vi "Calculation.vi"(4 "Calibration Factor":dbl, 5 "Frequency (Hz)":dbl, 6 "dµ (µg/mm)":dbl, 7 "t < 1.5 s ?":bool, 8 "dL (mm)":dbl, 9 "df (Hz)":dbl, 10 "Wire Linear Density In":dbl, 11 "Wire Length In":dbl) -> (0 "Linear Density (µm/mm)":dbl, 1 "Wire Length (mm)":dbl, 2 "dT (g)":dbl, 3 "Tension (g)":dbl)   [LabVIEW 2018]
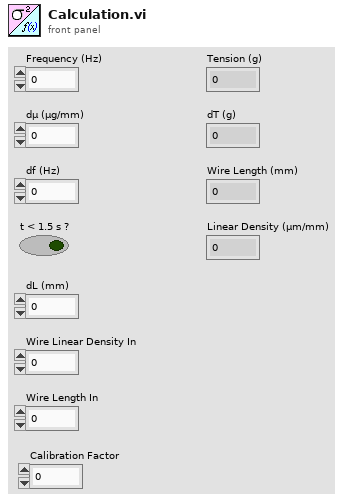
[diagram p1: front panel]
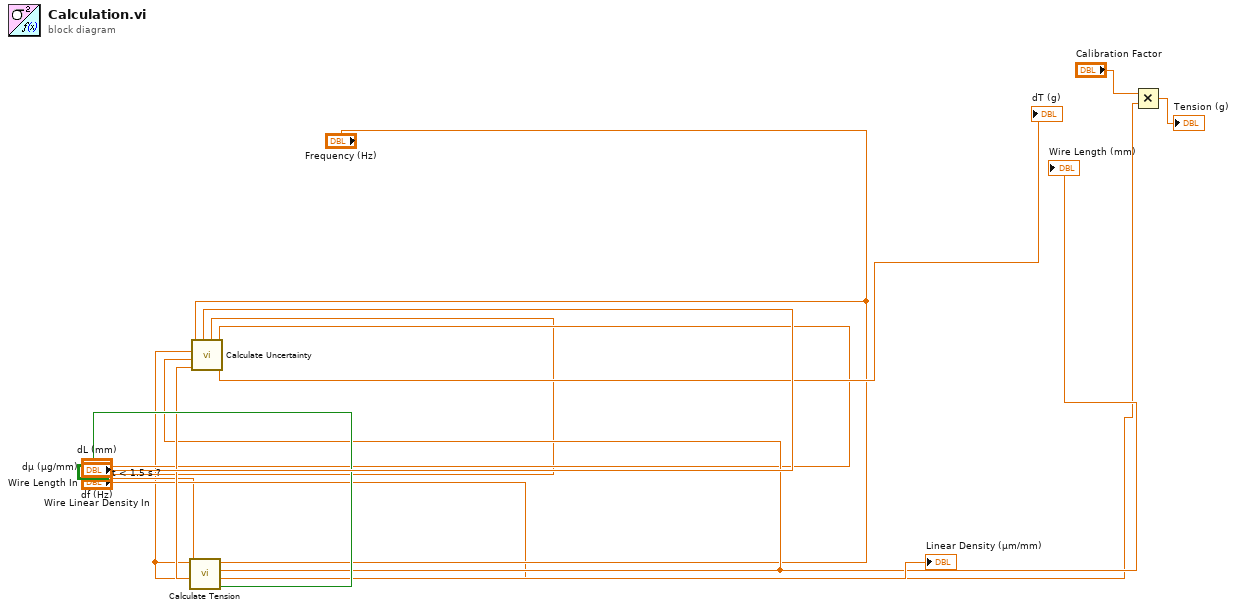
[diagram p0: block diagram]
diagram:
  n1 = call "Calculate Tension.vi"("t < X ?"="t < 1.5 s ?", "Wire Length"="Wire Length In", "Linear Density"="Wire Linear Density In", "Frequency"="Frequency (Hz)") -> ("Linear Density"=w11:dbl, "Wire Length"=w10:dbl, "Tension"=w1:dbl)  [unwired: 5 in]
  "Linear Density (µm/mm)" <- w11
  "Wire Length (mm)" <- w10
  n2 = call "Calculate Uncertainty.vi"("du"="dµ (µg/mm)", "dL"="dL (mm)", "df"="df (Hz)", "Linear Density"=w11, "Length"=w10, "Tension"=w1, "Frequency"="Frequency (Hz)") -> ("dT"=→"dT (g)":dbl)  [unwired: 4 in]
  n3 = Multiply(x="Calibration Factor", y=w1) -> (x*y=→"Tension (g)":dbl)
